vi "PathPlanner_ReplanningConfig_GetAll.vi"(11 "ReplanningConfig":T1) -> (0 "dynamicReplanningErrorSpikeThreshold":dbl=0.25, 1 "dynamicReplanningTotalErrorThreshold":dbl=1.0, 2 "enableDynamicReplanning":bool, 3 "enableInitialReplanning":bool=TRUE)   [LabVIEW 2019]
doc: "Get individual data elements from a PathPlanningConfig cluster\n\nInputs:\n - PathPlanningConfig - cluster\n\nOutputs:\n - EnableInitialReplanning - boolean Should the path be replanned at the start of path following if the robot is not already at the starting point?\n - EnableDynamicReplanning boolean - Should the path be replanned if the error grows too large or if a large error spike happens while following the path?\n - DynamicReplanningTotalErrorThreshold - double - The total error threshold, in meters, that will cause the path to be replanned\n - DynamicReplanningErrorSpikeThreshold - double - The error spike threshold, in meters, that will cause the path to be replanned"
uses:
  TypeDef/PathPlannerReplanningConfig.ctl
  PathPlanner24.lvlib
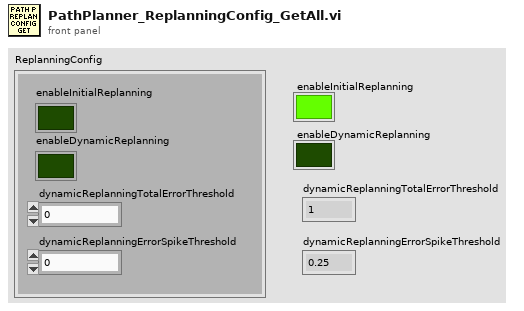
[diagram p1: front panel]
types:
  T1 = typedef "PathPlanner24.lvlib/PathPlannerReplanningConfig.ctl" = cluster{"enableInitialReplanning":bool, "enableDynamicReplanning":bool, "dynamicReplanningTotalErrorThreshold":dbl, "dynamicReplanningErrorSpikeThreshold":dbl}
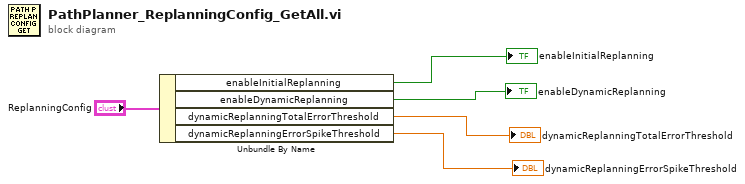
[diagram p0: block diagram]
diagram:
  n1 = Unbundle By Name("ReplanningConfig") -> ("enableInitialReplanning"=→"enableInitialReplanning":bool, "enableDynamicReplanning"=→"enableDynamicReplanning":bool, "dynamicReplanningTotalErrorThreshold"=→"dynamicReplanningTotalErrorThreshold":dbl, "dynamicReplanningErrorSpikeThreshold"=→"dynamicReplanningErrorSpikeThreshold":dbl)
